vi "zad5.vi"(8 "error in (no error)":errorcluster, 9 "Max":dbl, 10 "Min":dbl, 11 "Delta":dbl) -> (1 "error out":errorcluster, 2 "Array":dbl[](array[numeric]))   [LabVIEW 2017]
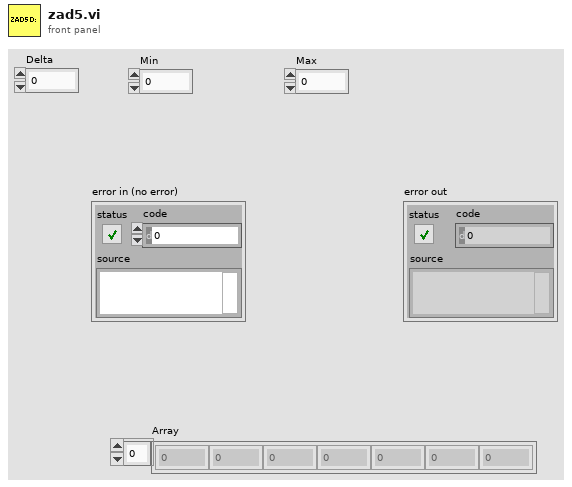
[diagram p1: front panel]
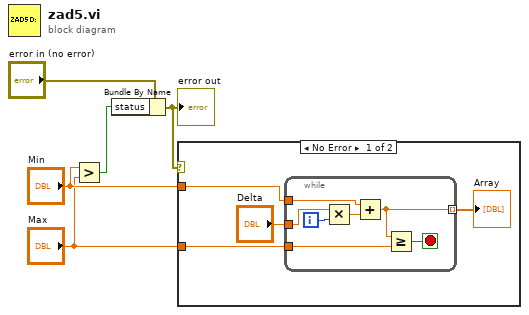
[diagram p0: block diagram]
diagram:
  n1 = Greater?(x="Min", y="Max") -> (0:w4:bool)
  n2 = Bundle By Name(cluster="error in (no error)", "status"=w4) -> (w3:errorcluster)
  "error out" <- w3
  n3 = case shown="No Error" w3 {
    tunnel: "Min" -> [w8 _]
    tunnel: "Max" -> [w7 _]
    frame No Error {
      n4 = while {
        tunnel: "Delta" -> [w16]
        tunnel: w8 -> [w13]
        tunnel: w7 -> [w12]
        tunnel: [w11] -> w6 mode=indexing
        i -> [w10]
        stop <- w14 stop-if-true
        n5 = Multiply(x=w16, y=w10) -> (x*y=w15:dbl)
        n6 = Add(x=w13, y=w15) -> (x+y=w11:dbl)
        n7 = Greater Or Equal?(x=w11, y=w12) -> (x >= y?=w14:bool)
      }
      "Array" <- w6
    }
    frame Error {
    }
  }
